vi "Min-Max Adjustable Boolean Counter.vi"(5 "Reset":bool, 6 "Dec Amount":dbl=1.0, 7 "Inc Amount":dbl=1.0, 8 "Decrease":bool, 9 "Increase":bool, 10 "Minimum":dbl=-1.0, 11 "Maximum":dbl=1.0) -> (1 "Counter":dbl)   [LabVIEW 2013]
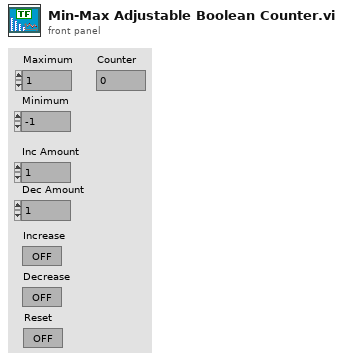
[diagram p1: front panel]
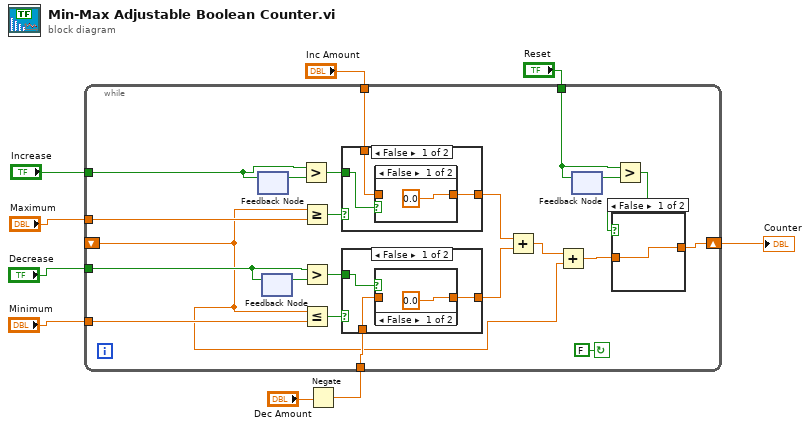
[diagram p0: block diagram]
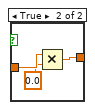
[diagram p2: hidden frame]
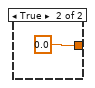
[diagram p4: hidden frame]
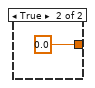
[diagram p6: hidden frame]
diagram:
  n1 = Negate(x="Dec Amount") -> (-x=w4:dbl)
  n2 = while {
    shift-right: [w14] -> w9
    shift-left: _ -> [w16]
    tunnel: "Increase" -> [w22]
    tunnel: "Maximum" -> [w21]
    tunnel: "Decrease" -> [w20]
    tunnel: "Minimum" -> [w19]
    tunnel: w4 -> [w18]
    tunnel: "Inc Amount" -> [w17]
    tunnel: "Reset" -> [w10]
    stop <- FALSE continue-if-true
    n3 = feedback-in #1(w22) -> ()
    n4 = feedback #1() -> (w25:bool)  [unwired: 1 in]
    n5 = feedback #2() -> (w24:bool)  [unwired: 1 in]
    n6 = feedback-in #2(w20) -> ()
    n7 = Greater?(x=w22, y=w25) -> (0:w31:bool)
    n8 = Greater Or Equal?(x=w16, y=w21) -> (x >= y?=w30:bool)
    n9 = Greater?(x=w20, y=w24) -> (0:w28:bool)
    n10 = Less Or Equal?(x=w16, y=w19) -> (x <= y?=w26:bool)
    n11 = case shown="False" w30 {
      tunnel: w31 -> [w44 _]
      tunnel: [w43 0.0] -> w29
      tunnel: w17 -> [w42 _]
      frame False {
        n12 = case shown="False" w44 {
          tunnel: [0.0 w46] -> w43
          tunnel: w42 -> [_ w46]
          frame False {
          }
          frame True {
          }
        }
      }
      frame True {
      }
    }
    n13 = case shown="False" w26 {
      tunnel: w28 -> [w38 _]
      tunnel: [w37 0.0] -> w27
      tunnel: w18 -> [w36 _]
      frame False {
        n14 = case shown="False" w38 {
          tunnel: [0.0 w40] -> w37
          tunnel: w36 -> [_ w40]
          frame False {
          }
          frame True {
          }
        }
      }
      frame True {
      }
    }
    n15 = Add(x=w29, y=w27) -> (x+y=w23:dbl)
    n16 = Add(x=w23, y=w16) -> (x+y=w15:dbl)
    n17 = feedback #3() -> (w13:bool)  [unwired: 1 in]
    n18 = feedback-in #3(w10) -> ()
    n19 = Greater?(x=w10, y=w13) -> (0:w12:bool)
    n20 = case shown="False" w12 {
      tunnel: w15 -> [w32 w35]
      tunnel: [w32 w33] -> w14
      frame False {
      }
      frame True {
        n21 = Multiply(x=w35, y=0.0) -> (x*y=w33:dbl)
      }
    }
  }
  "Counter" <- w9
